vi "Refresh GUI.vi"(8 "error in (no error)":errorcluster, 11 "Cfg Grandmaster in":refnum<class "Cfg Grandmaster.lvclass">) -> (0 "error out":errorcluster, 3 "Cfg Grandmaster out":refnum<class "Cfg Grandmaster.lvclass">)   [LabVIEW 2018, in "Configuration Grandmaster.lvlib" / "Cfg Grandmaster.lvclass"]
uses:
  Cfg Grandmaster.lvclass
  Cfg Grandmaster.lvclass/Cfg Grandmaster.ctl
  Common/Controls/TE_Designator.ctl
  Class Chassis Cfg/ChassisCfg.lvclass/ChassisCfg.ctl
  Class Chassis Cfg/Read GlobalBlockSize.vi
  Class Chassis Cfg/ChassisCfg.lvclass
  Class Timing Group/TimingGrp.lvclass
  Class FP Ctrls/FP Controls.lvclass
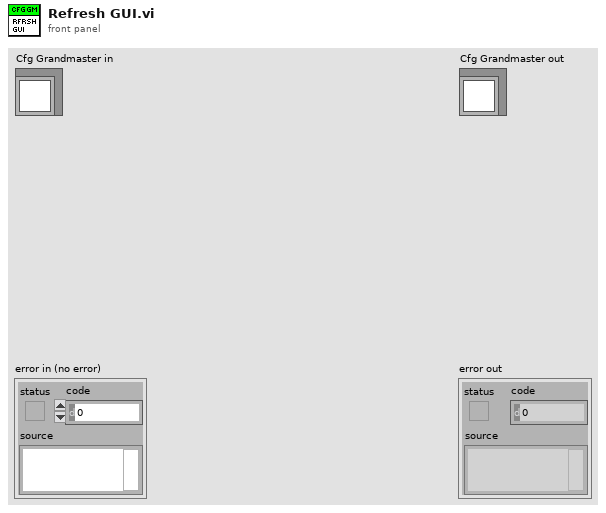
[diagram p1: front panel]
types:
  T1 = typedef "Selected Group.ctl" = cluster{"ChanGroup":i32, "Rate Class":T2}
  T2 = typedef "TE_Designator.ctl" = enum16{"High Speed", "Low Speed"}
  T3 = typedef "ge_Cfg wChassis.ctl" = cluster{"Chassis BOM":refnum<class "Chassis BOM.lvclass">, "Chassis Cfg":refnum<class "ChassisCfg.lvclass">, "Chassis Tasks":refnum<class "Chassis Tasks.lvclass">, "HW Error":bool, "Unsvd Chgs?":bool}
  T4 = typedef "DAQMan Mode.ctl" = enum16{"Cfg", "Run", "Shutting Down"}
  T5 = typedef "Group Timing Info.ctl" = cluster{"Rate":dbl, "ReadBlk":i32}
  T6 = typedef "LS Lock Sizes.ctl" = enum16{"No", "250ms", "500ms", "1s"}
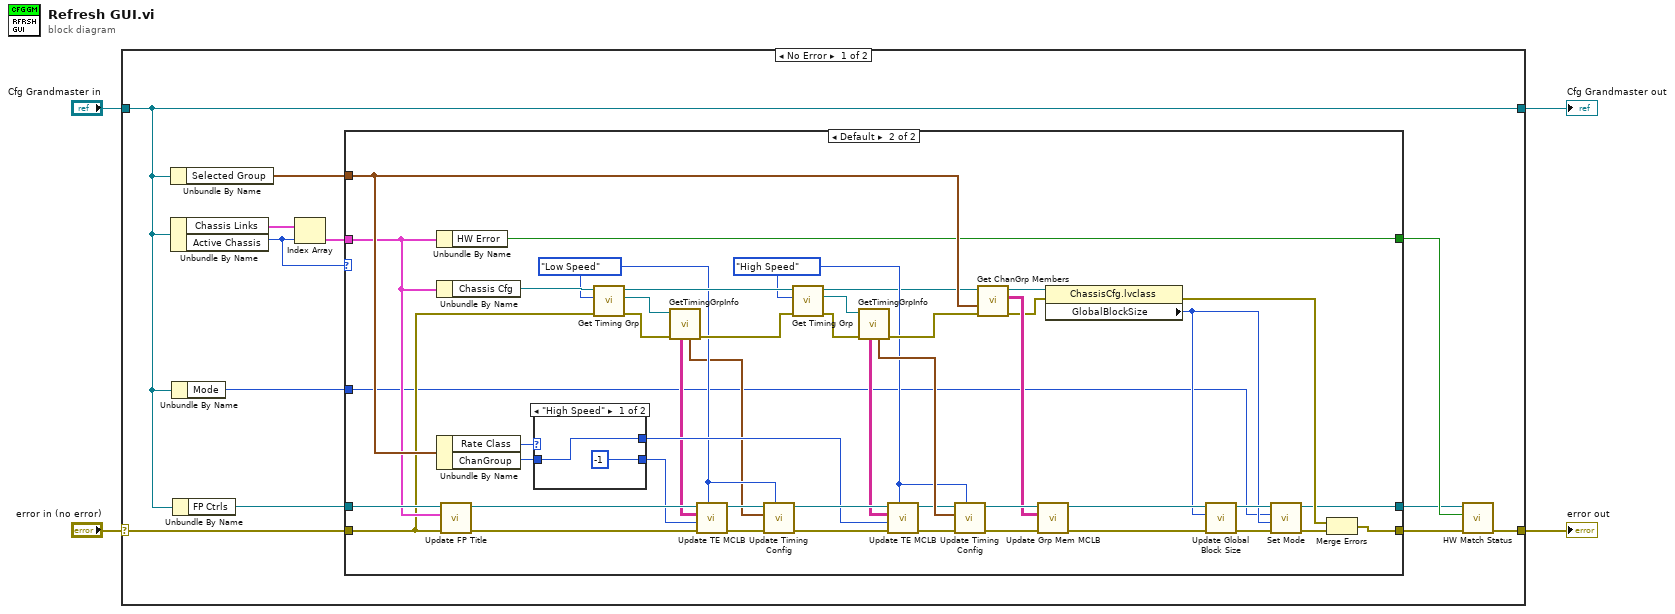
[diagram p0: block diagram]
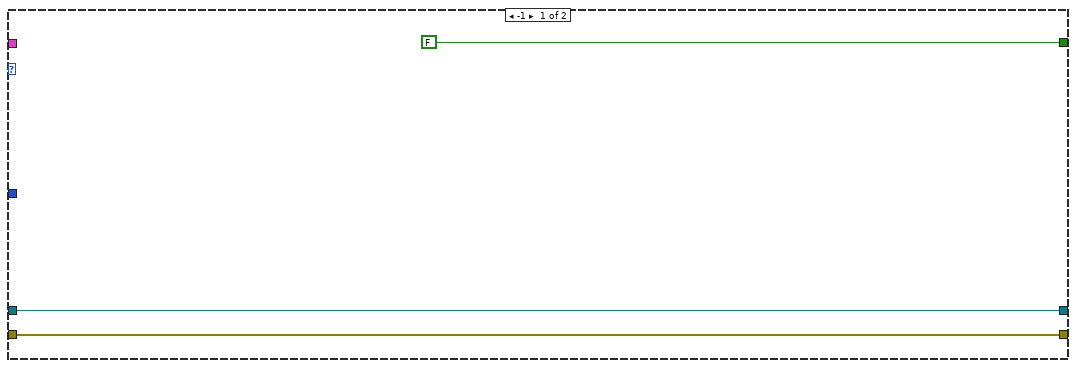
[diagram p2: hidden frame]
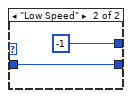
[diagram p3: hidden frame]
diagram:
  n1 = case shown="No Error" "error in (no error)" {
    selector: "error in (no error)" -> [w15 w72]
    tunnel: [w9 w72] -> w3
    tunnel: [w6 w71] -> w1
    tunnel: "Cfg Grandmaster in" -> [w6 w71]
    frame No Error {
      n2 = Unbundle By Name(w6) -> ("Selected Group"=w11:T1)
      n3 = Unbundle By Name(w6) -> ("Chassis Links"=w14:T3[], "Active Chassis"=w13:i32)
      n4 = Unbundle By Name(w6) -> ("Mode"=w5:T4)
      n5 = Unbundle By Name(w6) -> ("FP Ctrls"=w12:refnum<class "FP Controls.lvclass">)
      n6 = Index Array(array=w14, index=w13) -> (element=w16:T3)
      n7 = case shown="Default" w13 {
        tunnel: w15 -> [w19 w42]
        tunnel: w11 -> [_ w64]
        tunnel: [w19 w43] -> w10
        tunnel: w16 -> [_ w60]
        tunnel: [FALSE ("HW Error") w63] -> w8
        tunnel: w12 -> [w17 w61]
        tunnel: [w17 w22] -> w7
        tunnel: w5 -> [_ w20]
        frame -1 {
        }
        frame Default {
          w44 = TE_Designator."High Speed" ("Timing Engine")
          w45 = TE_Designator."Low Speed" ("Timing Engine")
          n8 = Unbundle By Name(w60) -> ("HW Error"=w63:bool)
          n9 = Unbundle By Name(w60) -> ("Chassis Cfg"=w62:refnum<class "ChassisCfg.lvclass">)
          n10 = Unbundle By Name(w64) -> ("Rate Class"=w66:T2, "ChanGroup"=w65:i32)
          n11 = call "Update FP Title.vi"("error in (no error)"=w42, "Cfg wChassis"=w60, "FP Controls in"=w61) -> ("error out"=w48:errorcluster, "FP Controls out"=w49:refnum<class "FP Controls.lvclass">)  [unwired: 7 in]
          n12 = case shown="\"High Speed\"" w66 {
            tunnel: w65 -> [w68 w70]
            tunnel: [w68 -1 ("ChanGroup")] -> w52
            tunnel: [-1 ("ChanGroup") w70] -> w47
            frame "High Speed" {
            }
            frame "Low Speed" {
            }
          }
          n13 = call "Get Timing Grp.vi"("error in (no error)"=w42, "Timing Engine"=w45, "Chassis Cfg"=w62) -> ("error out"=w40:errorcluster, "Timing Groups"=w41:refnum<class "TimingGrp.lvclass">, "Chassis Cfg"=w58:refnum<class "ChassisCfg.lvclass">)  [unwired: 6 in]
          n14 = call "GetTimingGrpInfo.vi"("error in"=w40, "TimingGrp in"=w41) -> ("error out"=w57:errorcluster, "Timing Cfg"=w38:T5, "Grp List"=w39:string[][])  [unwired: 4 in, 3 out]
          n15 = call "Update TE MCLB.vi"("TimingEngine"=w45, "error in"=w48, "Selected Row"=w47, "Item Names"=w39, "FP Ctrls"=w49) -> ("error out"=w50:errorcluster, "FP Ctrls"=w51:refnum<class "FP Controls.lvclass">)  [unwired: 5 in]
          n16 = call "Update Timing Config.vi"("Timing Engine"=w45, "error in (no error)"=w50, "Timing Cfg"=w38, "FP Controls in"=w51) -> ("error out"=w53:errorcluster, "FP Controls out"=w54:refnum<class "FP Controls.lvclass">)  [unwired: 6 in]
          n17 = call "Get Timing Grp.vi"("error in (no error)"=w57, "Timing Engine"=w44, "Chassis Cfg"=w58) -> ("error out"=w36:errorcluster, "Timing Groups"=w37:refnum<class "TimingGrp.lvclass">, "Chassis Cfg"=w29:refnum<class "ChassisCfg.lvclass">)  [unwired: 6 in]
          n18 = call "GetTimingGrpInfo.vi"("error in"=w36, "TimingGrp in"=w37) -> ("error out"=w46:errorcluster, "Timing Cfg"=w59:T5, "Grp List"=w35:string[][])  [unwired: 4 in, 3 out]
          n19 = call "Update TE MCLB.vi"("TimingEngine"=w44, "error in"=w53, "Selected Row"=w52, "Item Names"=w35, "FP Ctrls"=w54) -> ("error out"=w55:errorcluster, "FP Ctrls"=w56:refnum<class "FP Controls.lvclass">)  [unwired: 5 in]
          n20 = call "Update Timing Config.vi"("Timing Engine"=w44, "error in (no error)"=w55, "Timing Cfg"=w59, "FP Controls in"=w56) -> ("error out"=w34:errorcluster, "FP Controls out"=w33:refnum<class "FP Controls.lvclass">)  [unwired: 6 in]
          n21 = call "Get ChanGrp Members.vi"("error in"=w46, "Channel Groups"=w64, "Chassis Cfg"=w29) -> ("error out"=w27:errorcluster, "Group Members"=w32:string[][], "Chassis Cfg"=w28:refnum<class "ChassisCfg.lvclass">)  [unwired: 6 in]
          n22 = call "Update Grp Mem MCLB.vi"("error in"=w34, "Item Names"=w32, "FP Ctrls"=w33) -> ("error out"=w30:errorcluster, "FP Ctrls"=w31:refnum<class "FP Controls.lvclass">)  [unwired: 7 in]
          n23 = property class="ChassisCfg.lvclass"(reference=w28, error in=w27) -> (error out=w26:errorcluster, "GlobalBlockSize"=w23:T6)  [unwired: 1 out]
          n24 = call "Update Global Block Size.vi"("error in (no error)"=w30, "LockToLS"=w23, "FP Controls in"=w31) -> ("error out"=w25:errorcluster, "FP Controls out"=w24:refnum<class "FP Controls.lvclass">)  [unwired: 7 in]
          n25 = call "Set Mode.vi"("error in (no error)"=w25, "LockToLS"=w23, "Mode"=w20, "FP Controls in"=w24) -> ("error out"=w21:errorcluster, "FP Controls out"=w22:refnum<class "FP Controls.lvclass">)  [unwired: 6 in]
          n26 = Merge Errors(w26, w21) -> (w43:errorcluster)
        }
      }
      n27 = call "HW Match Status.vi"("error in (no error)"=w10, "Pass (F) / Fail (T)"=w8, "FP Controls in"=w7) -> ("error out"=w9:errorcluster)  [unwired: 7 in, 1 out]
    }
    frame Error {
    }
  }
  "error out" <- w3
  "Cfg Grandmaster out" <- w1
